vi "reset_sp6_link.vi"(8 "error in (no error)":errorcluster, 11 "address":string="10.3.173.11") -> (0 "error out":errorcluster)   [LabVIEW 2017]
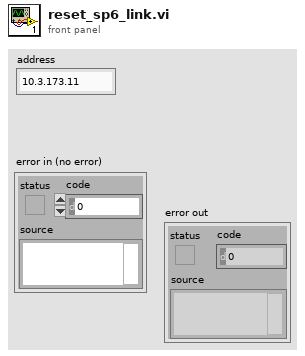
[diagram p1: front panel]
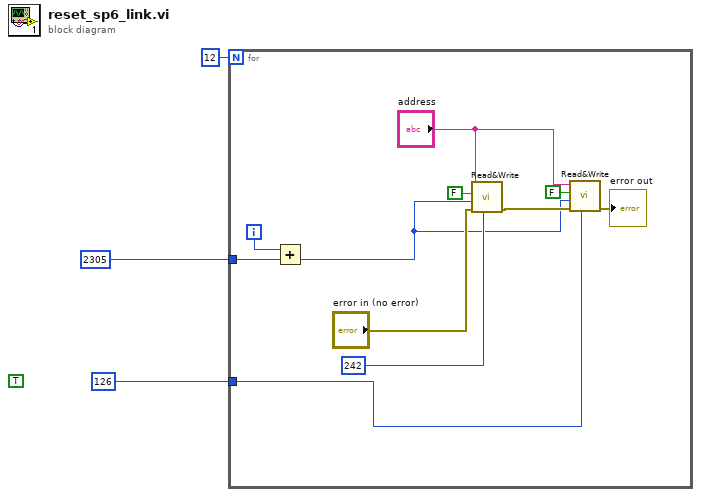
[diagram p0: block diagram]
diagram:
  (unwired) TRUE
  n1 = for {
    N: 12 -> [_]
    tunnel: u32 2305 ("Address") -> [w7]
    tunnel: u8 126 ("In 3") -> [w6]
    i -> [w4]
    n2 = Add(x=w4, y=w7) -> (x+y=w5:u32)
    n3 = call "Read&Write.vi"("In"=u8 242, "error in (no error)"="error in (no error)", "Address"=w5, "Read (TRUE)"=FALSE, "address"="address") -> ("error out"=w14:errorcluster)  [unwired: 5 in, 1 out]
    n4 = call "Read&Write.vi"("In"=w6, "error in (no error)"=w14, "Address"=w5, "Read (TRUE)"=FALSE, "address"="address") -> ("error out"=→"error out":errorcluster)  [unwired: 5 in, 1 out]
  }
